vi "Dequeue Incoming Command.vi"(8 "Error In":errorcluster, 11 "Process In":refnum<class "Process.lvclass">) -> (0 "Error Out":errorcluster, 2 "Process Message":T1, 3 "Process Out":refnum<class "Process.lvclass">)   [LabVIEW 2019, in "Process.lvclass"]
uses:
  Process.lvclass
  Public/Controls/Process Message.ctl
  Accessors/Message Queue/Get Message Queue.vi
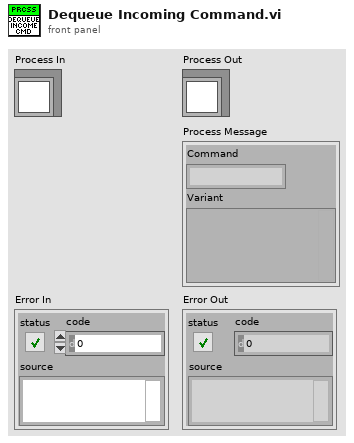
[diagram p1: front panel]
types:
  T1 = typedef "Process.lvclass/Process Message.ctl" = cluster{"Command":string, "Variant":variant}
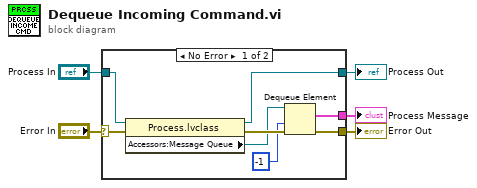
[diagram p0: block diagram]
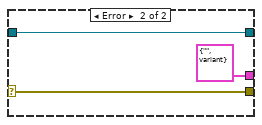
[diagram p2: hidden frame]
diagram:
  n1 = case shown="No Error" "Error In" {
    selector: "Error In" -> [w13 w16]
    tunnel: [w6 w16] -> w4
    tunnel: "Process In" -> [w12 w15]
    tunnel: [w8 w15] -> w2
    tunnel: [w7 T1 {"Command"="", "Variant"=variant} ("Process Message")] -> w1
    frame No Error {
      n2 = property class="Process.lvclass"(reference=w12, error in=w13) -> (reference out=w8:refnum<class "Process.lvclass">, error out=w11:errorcluster, "Accessors:Message Queue"=w10:refnum<queue>)
      n3 = Dequeue Element(queue=w10, timeout in ms (-1)=-1, error in (no error)=w11) -> (element=w7:T1, error out=w6:errorcluster)  [unwired: 2 out]
    }
    frame Error {
    }
  }
  "Process Out" <- w2
  "Error Out" <- w4
  "Process Message" <- w1
